vi "simula ai.vi"(11 "ARRAY SIM AI":cluster{"Amplitude":dbl, "Precision %":dbl}[](array[cluster])) -> (3 "Array":dbl[](array[numeric]))   [LabVIEW 2019]
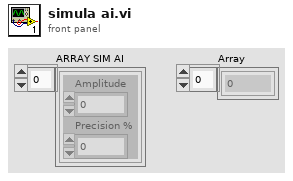
[diagram p1: front panel]
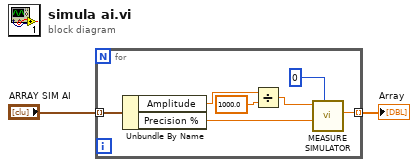
[diagram p0: block diagram]
diagram:
  n1 = for {
    tunnel: "ARRAY SIM AI" -> [w8] mode=indexing
    tunnel: [w6] -> w2 mode=indexing
    n2 = Unbundle By Name(w8) -> ("Amplitude"=w5:dbl, "Precision %"=w7:dbl)
    n3 = Divide(x=w5, y=1000.0) -> (x/y=w3:dbl)
    n4 = call <userlib>:"MEASURE SIMULATOR.vi"("delay (100)"=u32 0, "precision %"=w7, "amplitude"=w3) -> ("value"=w6:dbl)  [unwired: 8 in]
  }
  "Array" <- w2
